vi "BRig_dataLC_ENL2_PostR_Count_l1.vi"() -> (2 "output_ENL2_PostR_Count":i32)   [LabVIEW 2014]
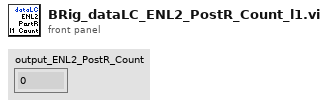
[diagram p1: front panel]
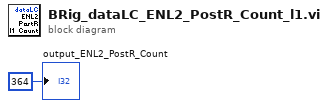
[diagram p0: block diagram]
diagram:
  "output_ENL2_PostR_Count" <- 364 ("output_iBlock")
